vi "Parse Array.vi"(8 "error in (no error)":errorcluster, 9 "Level":u32, 11 "String":string) -> (0 "error out":errorcluster, 2 "Value":variant[](array[variant]), 3 "Remaining String":string)   [LabVIEW 2015, in "YAML Parser.lvclass"]
uses:
  YAML Parser.lvclass
panel:
  out "First Letter":string
  out "String en Cours d'Analyse":string
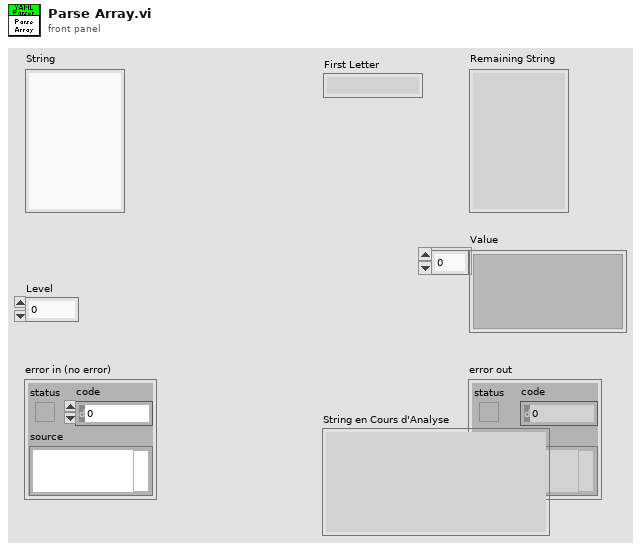
[diagram p1: front panel]
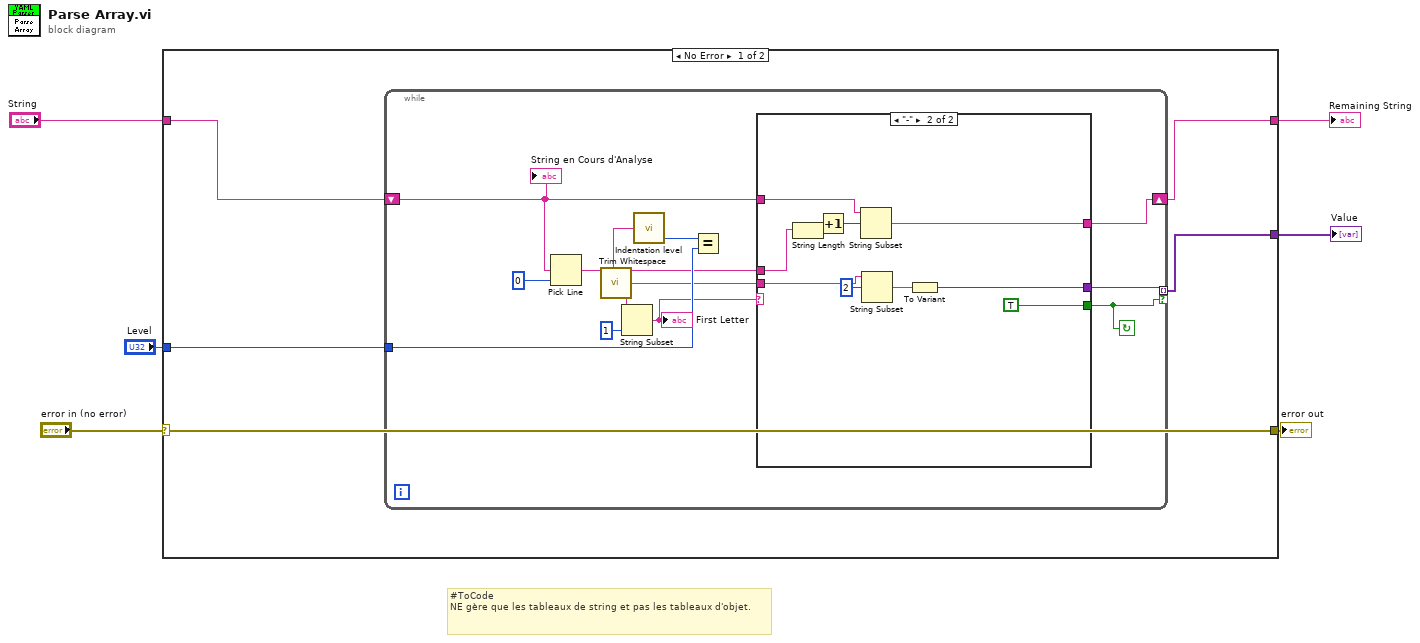
[diagram p0: block diagram]
diagram:
  # "#ToCode\nNE gère que les tableaux de string et pas les tableaux d'objet."
  n1 = case shown="No Error" "error in (no error)" {
    selector: "error in (no error)" -> [w11 w36]
    tunnel: [w11 w36] -> w5
    tunnel: "String" -> [w10 w35]
    tunnel: [w8 w35] -> w3
    tunnel: "Level" -> [w9 _]
    tunnel: [w7 _] -> w1
    frame No Error {
      n2 = while {
        tunnel: w9 -> [w19]
        shift-right: [w13] -> w8
        shift-left: w10 -> [w14]
        tunnel: [w16] -> w7 mode=indexing if=w15
        stop <- w15 continue-if-true
        n3 = Pick Line(multi-line string=w14, line index=0) -> (output string=w12:string)  [unwired: 1 in]
        n4 = call <vilib>:"Trim Whitespace.vi"("string"=w12) -> ("trimmed string"=w17:string)  [unwired: 1 in]
        n5 = String Subset(string=w17, length (rest)=1 ("length (rest)")) -> (substring=w18:string)  [unwired: 1 in]
        "First Letter" <- w18
        n6 = call "Indentation level.vi"("String"=w12) -> ("Level"=w20:u32)  [unwired: 2 out]
        n7 = Equal?(x=w20, y=w19) -> ()  [unwired: 1 out]
        n8 = case shown="\"-\"" w18 {
          tunnel: w17 -> [w24 w34]
          tunnel: [w24 w25] -> w16
          tunnel: [_ TRUE] -> w15
          tunnel: w14 -> [w23 w30]
          tunnel: [w23 w29] -> w13
          tunnel: w12 -> [_ w28]
          frame Default {
          }
          frame "-" {
            n9 = String Length(string=w28) -> (length=w27:i32)
            n10 = Increment(x=w27) -> (x+1=w26:i32)
            n11 = String Subset(string=w30, offset (0)=w26) -> (substring=w29:string)  [unwired: 1 in]
            n12 = String Subset(string=w34, offset (0)=2) -> (substring=w32:string)  [unwired: 1 in]
            n13 = To Variant(anything=w32) -> (Variant=w25:variant)
          }
        }
        "String en Cours d'Analyse" <- w14
      }
    }
    frame Error {
    }
  }
  "error out" <- w5
  "Value" <- w1
  "Remaining String" <- w3
